vi "About.vi"   [LabVIEW 2020]
panel:
  # "CaseSelect"
  # "is a plugin for the JKI Right-Click Framework.  You can \nfind more information and participate in the discussion\nat"
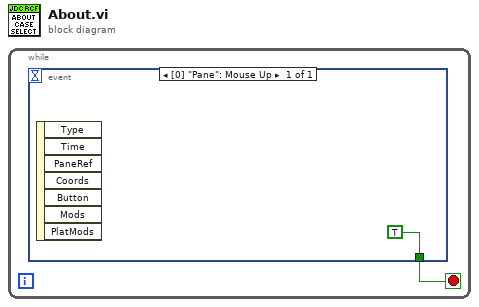
[diagram p0: block diagram]
diagram:
  n1 = while {
    stop <- w1 stop-if-true
    n2 = event shown="[0] \"Pane\": Mouse Up" {
      selector: _ -> [_]
      dyn-events: _ -> [_]
      timeout: _ -> [_]
      tunnel: [TRUE] -> w1
      event Mouse Up {
        n3 = event-data() -> ()  [unwired: 8 out]
      }
    }
  }
